vi "TCPIPmain.vi"(6 "data":T1(array[cluster]), 7 "config":T2, 8 "error in":errorcluster, 9 "data in":string, 10 "targer":enum16{"主舱外回路", "主舱内回路", "实验舱外回路", "实验舱内回路"}(ring), 11 "Enum":T3) -> (0 "error out":errorcluster, 1 "LED":bool[](array[boolean]), 2 "data out":T1(array[cluster]), 3 "Data?":bool[](array[boolean]))   [LabVIEW 2011]
uses:
  TCPIP_enum.ctl
  TCPIPconfig.ctl
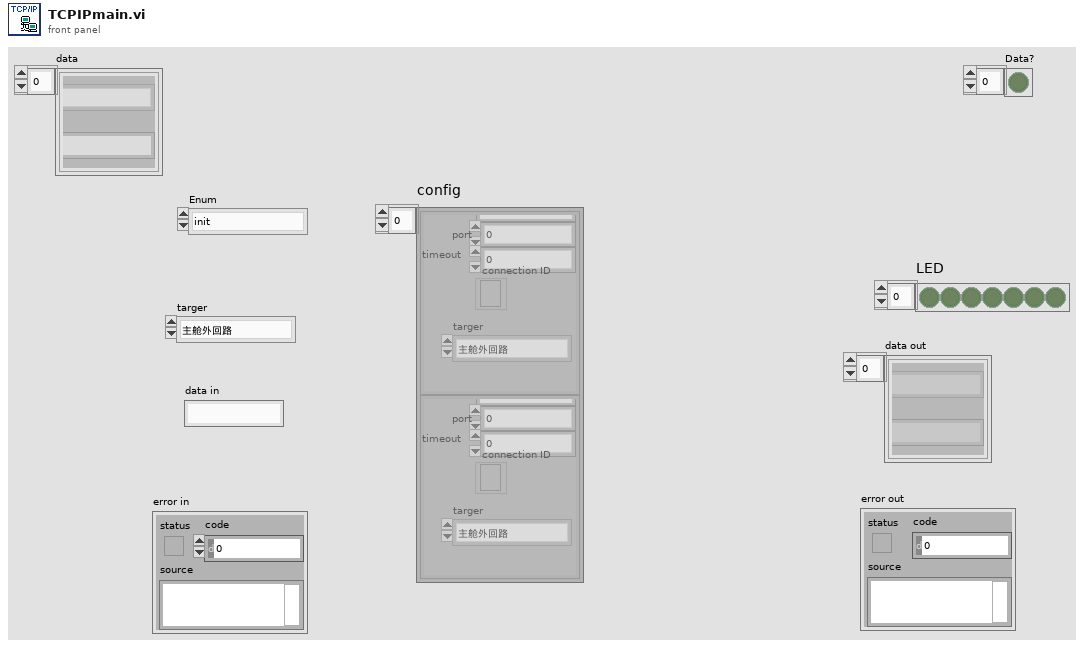
[diagram p1: front panel]
types:
  T1 = cluster{"targer":enum16{"主舱外回路", "主舱内回路", "实验舱外回路", "实验舱内回路"}, "data":string}[]
  T2 = typedef "TCPIPconfig.ctl" = cluster{"add":string, "port":u32, "timeout":u16, "connection ID":refnum<k5>, "targer":enum16{"主舱外回路", "主舱内回路", "实验舱外回路", "实验舱内回路"}}[]
  T3 = typedef "TCPIP_enum.ctl" = enum16{"init", "connect", "command", "write", "read", "close", "null"}
  T4 = cluster{"targer":enum16{"主舱外回路", "主舱内回路", "实验舱外回路", "实验舱内回路"}, "data":string}
  T5 = cluster{"add":string, "port":u32, "timeout":u16, "connection ID":refnum<k5>, "targer":enum16{"主舱外回路", "主舱内回路", "实验舱外回路", "实验舱内回路"}}
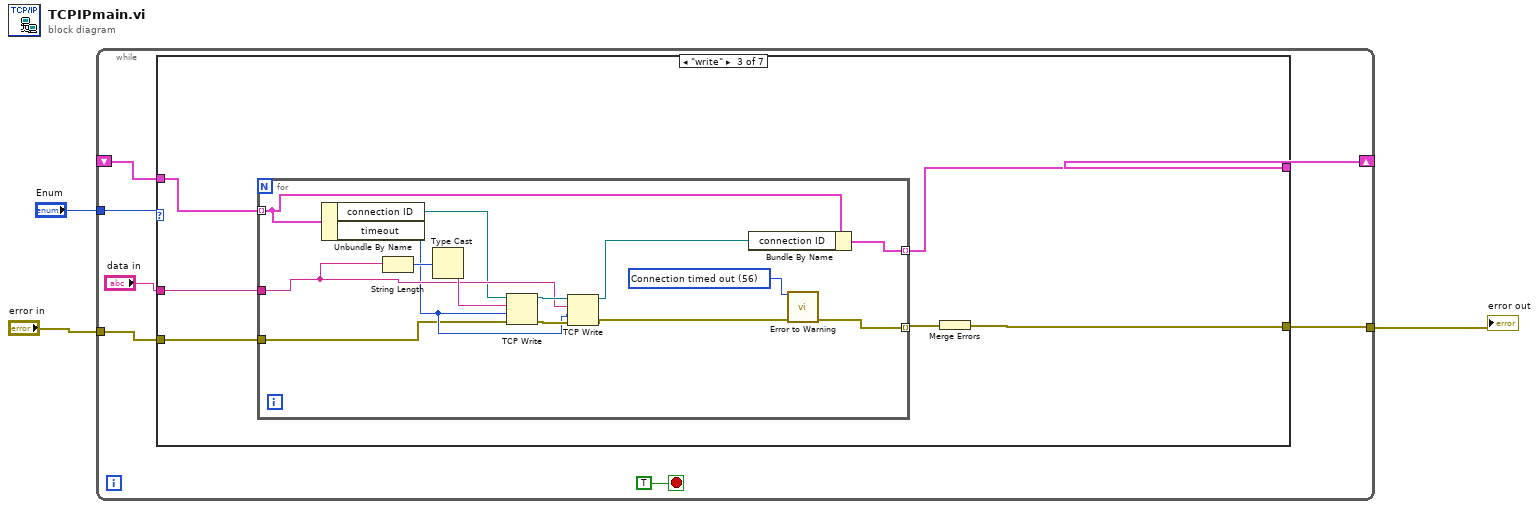
[diagram p0: block diagram]
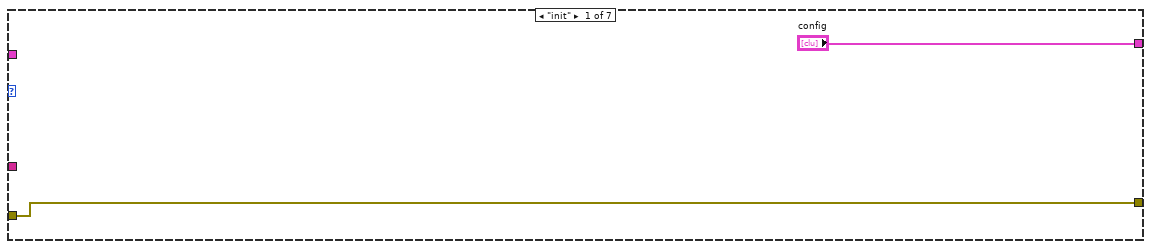
[diagram p2: hidden frame]
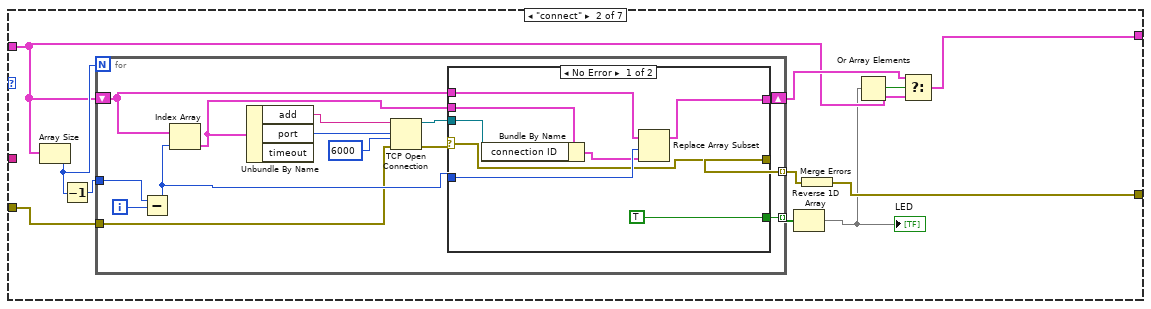
[diagram p3: hidden frame]
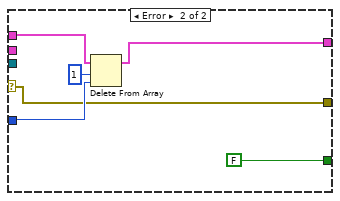
[diagram p4: hidden frame]
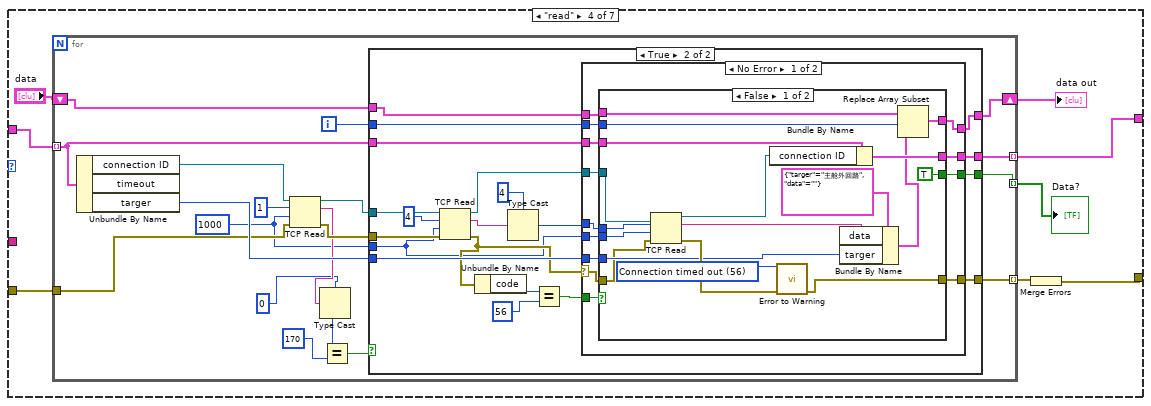
[diagram p5: hidden frame]
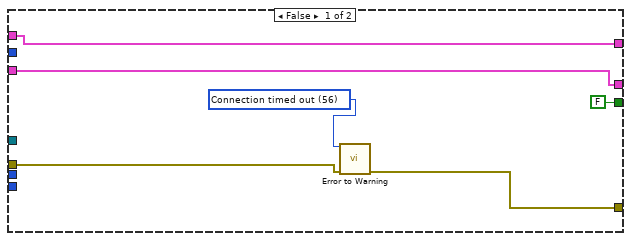
[diagram p6: hidden frame]
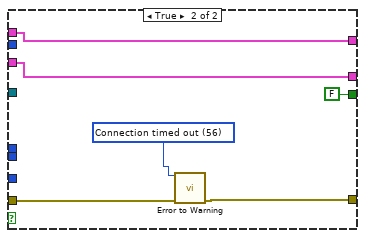
[diagram p7: hidden frame]
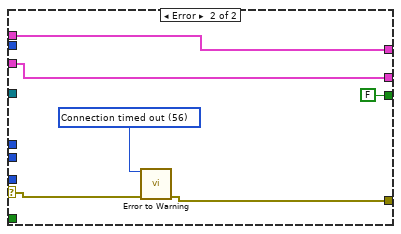
[diagram p8: hidden frame]
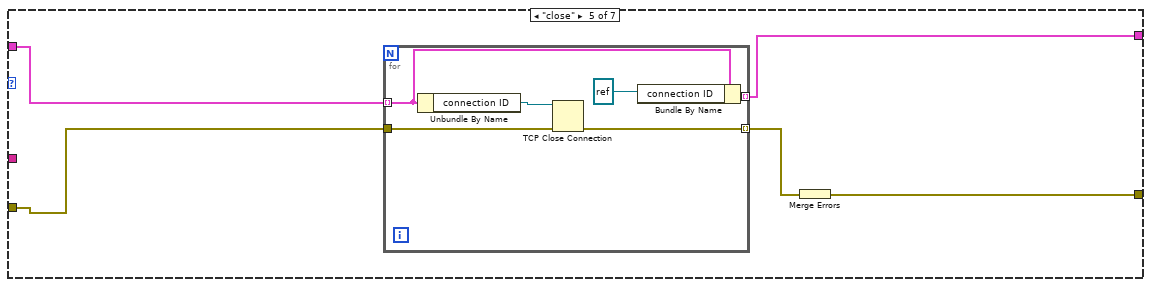
[diagram p9: hidden frame]
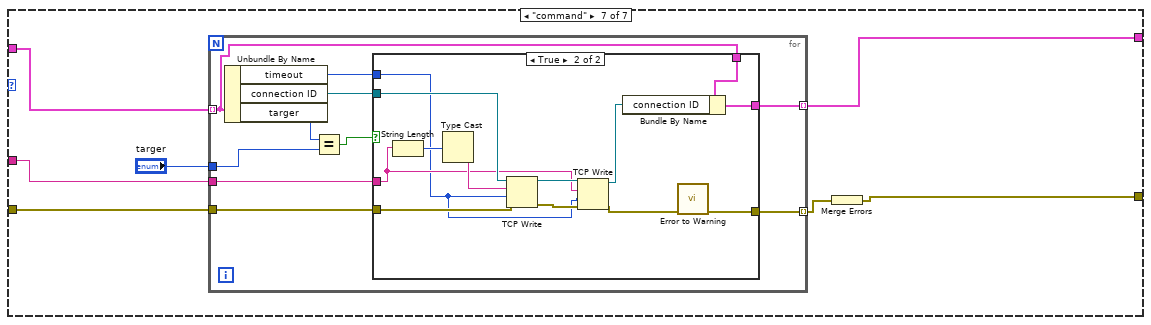
[diagram p11: hidden frame]
diagram:
  n1 = while {
    shift-right: [w8] -> _
    shift-left: _ -> [w7]
    tunnel: [w6] -> w2
    tunnel: "error in" -> [w5]
    tunnel: "Enum" -> [w9]
    stop <- TRUE stop-if-true
    n2 = case shown="\"write\"" w9 {
      tunnel: ["config" w14 w56 w78 w168 w180 w183] -> w8
      tunnel: w7 -> [_ w15 w57 w79 w172 w180 w187]
      tunnel: [w11 w20 w54 w76 w169 w179 w182] -> w6
      tunnel: w5 -> [w11 w22 w53 w75 w171 w179 w185]
      tunnel: "data in" -> [_ _ w52 _ _ _ w184]
      frame "init" {
      }
      frame "connect" {
        n3 = Array Size(array=w15) -> (size(s)=w19:i32)
        n4 = Decrement(x=w19) -> (x-1=w23:i32)
        n5 = for {
          N: w19 -> [_]
          shift-right: [w29] -> w16
          shift-left: w15 -> [w33]
          tunnel: w23 -> [w31]
          tunnel: w22 -> [w28]
          tunnel: [w27] -> w21 mode=indexing
          tunnel: [w26] -> w18 mode=indexing
          i -> [w32]
          n6 = Subtract(x=w31, y=w32) -> (x-y=w30:i32)
          n7 = Index Array(array=w33, index=w30) -> (element=w34:T5)
          n8 = Unbundle By Name(w34) -> ("add"=w37:string, "port"=w25:u32)  [unwired: 1 out]
          n9 = TCP Open Connection(address=w37, remote port or service name=w25, timeout ms (60000)=6000, error in (no error)=w28) -> (connection ID=w36:refnum<k5>, error out=w35:errorcluster)  [unwired: 1 in]
          n10 = case shown="No Error" w35 {
            selector: w35 -> [w39 w47]
            tunnel: w36 -> [w45 _]
            tunnel: w34 -> [w44 _]
            tunnel: w33 -> [w43 w51]
            tunnel: w30 -> [w42 w49]
            tunnel: [w40 w48] -> w29
            tunnel: [w39 w47] -> w27
            tunnel: [TRUE FALSE] -> w26
            frame No Error {
              n11 = Bundle By Name(cluster=w44, "connection ID"=w45) -> (w41:T5)
              n12 = Replace Array Subset "Replace Array Subset"(array=w43, new element=w41, index=w42) -> (w40:T2)
            }
            frame Error {
              n13 = Delete From Array(array=w51, length=1, index=w49) -> (array with subset deleted=w48:T2)  [unwired: 1 out]
            }
          }
        }
        n14 = Reverse 1D Array(array=w18) -> (reversed array=w13:bool[])
        "LED" <- w13
        n15 = Merge Errors(w21) -> (w20:errorcluster)
        n16 = Or Array Elements(Boolean array=w13) -> (logical OR=w17:bool)
        n17 = Select(t=w16, s=w17, f=w15) -> (s? t:f=w14:T2)
      }
      frame "write" {
        n18 = for {
          tunnel: w57 -> [w63] mode=indexing
          tunnel: w52 -> [w66]
          tunnel: [w61] -> w56 mode=indexing
          tunnel: [w60] -> w55 mode=indexing
          tunnel: w53 -> [w59]
          w58 = 56 items=["No Error", "Argument Error", "Memory Full", "Out of Zone", "End of File", "File Already Open", "Generic File IO Error", "File Not Found", "File Permission Error", "Disk Full", "Duplicate Path", "Too Many Files Open", "Not Enabled", "Resource File Not Found", "Cannot Add Resource", "Resource Not Found", "Image Not Found", "Image Memory Error", "Pen Does Not Exist", "Config Bad Type", "Config Token Not Found", "Config Parse Error", "Config Memory Error", "Bad External Code Format", "Bad External Code Offset", "External Code Not Present", "Null Window", "Destroy Window Mixup", "Null Menu", "Print Aborted", "Bad Print Record", "Print Driver Error", "Windows Error During Print", "Memory Error During Print", "Print Dialog Error", "Generic Print Error", "Invalid Device Refnum", "Device Not Found", "Device Parameter Error", "Device Unit Error", "Can't Open Device", "Device Call Aborted", "Generic Error", "Cancelled By User", "Object ID Too Low", "Object ID Too High", "Object Not In Heap", "Unknown Heap", "Bad DefProc ID", "DefProc Not In Table", "Message Out Of Range", "Null Method", "Unknown Message", "Manager Call Not Supported", "Bad address", "Connection In progress", "Connection timed out", "Connection is already in progress", "Network attribute not supported", "Network error", "Address in use", "System out of memory", "Connection aborted", "Connection refused", "Connection is not connected", "Connection is already connected", "Connection closed", "Initialize error (interapplication manager)", "Bad occurrence", "Wait on unbound occurrence handler", "Occurrence queue overflow", "Bad path", "Semaphore not signaled", "Unrecognized type (interapplication manager)"] ("1st Error to Convert")
          n19 = Unbundle By Name(w63) -> ("connection ID"=w65:refnum<k5>, "timeout"=w64:u16)
          n20 = String Length(string=w66) -> (length=w71:i32)
          n21 = Type Cast(x=w71) -> (*(type *) &x=w68:string)  [unwired: 1 out]
          n22 = TCP Write(connection ID=w65, data in=w68, error in (no error)=w59, 9:w64) -> (connection ID out=w70:refnum<k5>, error out=w69:errorcluster)  [unwired: 1 out]
          n23 = TCP Write(connection ID=w70, data in=w66, error in (no error)=w69, 9:w64) -> (connection ID out=w62:refnum<k5>, error out=w67:errorcluster)  [unwired: 1 out]
          n24 = Bundle By Name(cluster=w63, "connection ID"=w62) -> (w61:T5)
          n25 = call <vilib>:"Error to Warning.vi"("1st Error to Convert"=w58, "error in"=w67) -> ("warning out"=w60:errorcluster)  [unwired: 4 in, 9 out]
        }
        n26 = Merge Errors(w55) -> (w54:errorcluster)
      }
      frame "read" {
        n27 = for {
          tunnel: w79 -> [w98] mode=indexing
          tunnel: [w97] -> w78 mode=indexing
          tunnel: [w96] -> w77 mode=indexing
          tunnel: w75 -> [w94]
          shift-right: [w83] -> w73
          shift-left: "data" -> [w84]
          tunnel: [w81] -> w72 mode=indexing
          i -> [w82]
          w80 = 1000 ("timeout ms (25000)")
          n28 = Unbundle By Name(w98) -> ("connection ID"=w93:refnum<k5>, "targer"=w95:enum16{"主舱外回路", "主舱内回路", "实验舱外回路", "实验舱内回路"})  [unwired: 1 out]
          n29 = TCP Read(connection ID=w93, bytes to read=1, error in (no error)=w94, 9:w80) -> (connection ID out=w90:refnum<k5>, data out=w89:string, error out=w91:errorcluster)  [unwired: 1 out]
          n30 = Type Cast(type=u8 0, x=w89) -> (*(type *) &x=w87:u8)
          n31 = Equal?(x=w87, y=u8 170) -> (x = y?=w85:bool)
          n32 = case shown="True" w85 {
            tunnel: w90 -> [_ w120]
            tunnel: w98 -> [w104 w119]
            tunnel: [w104 w118] -> w97
            tunnel: [w100 w117] -> w96
            tunnel: w91 -> [w101 w116]
            tunnel: w95 -> [_ w115]
            tunnel: w80 -> [_ w109]
            tunnel: w84 -> [w103 w108]
            tunnel: [w103 w107] -> w83
            tunnel: w82 -> [_ w106]
            tunnel: [FALSE w105] -> w81
            frame False {
              w99 = 56 items=["No Error", "Argument Error", "Memory Full", "Out of Zone", "End of File", "File Already Open", "Generic File IO Error", "File Not Found", "File Permission Error", "Disk Full", "Duplicate Path", "Too Many Files Open", "Not Enabled", "Resource File Not Found", "Cannot Add Resource", "Resource Not Found", "Image Not Found", "Image Memory Error", "Pen Does Not Exist", "Config Bad Type", "Config Token Not Found", "Config Parse Error", "Config Memory Error", "Bad External Code Format", "Bad External Code Offset", "External Code Not Present", "Null Window", "Destroy Window Mixup", "Null Menu", "Print Aborted", "Bad Print Record", "Print Driver Error", "Windows Error During Print", "Memory Error During Print", "Print Dialog Error", "Generic Print Error", "Invalid Device Refnum", "Device Not Found", "Device Parameter Error", "Device Unit Error", "Can't Open Device", "Device Call Aborted", "Generic Error", "Cancelled By User", "Object ID Too Low", "Object ID Too High", "Object Not In Heap", "Unknown Heap", "Bad DefProc ID", "DefProc Not In Table", "Message Out Of Range", "Null Method", "Unknown Message", "Manager Call Not Supported", "Bad address", "Connection In progress", "Connection timed out", "Connection is already in progress", "Network attribute not supported", "Network error", "Address in use", "System out of memory", "Connection aborted", "Connection refused", "Connection is not connected", "Connection is already connected", "Connection closed", "Initialize error (interapplication manager)", "Bad occurrence", "Wait on unbound occurrence handler", "Occurrence queue overflow", "Bad path", "Semaphore not signaled", "Unrecognized type (interapplication manager)"] ("1st Error to Convert")
              n33 = call <vilib>:"Error to Warning.vi"("1st Error to Convert"=w99, "error in"=w101) -> ("warning out"=w100:errorcluster)  [unwired: 4 in, 9 out]
            }
            frame True {
              n34 = TCP Read(connection ID=w120, bytes to read=4, error in (no error)=w116, 9:w109) -> (connection ID out=w123:refnum<k5>, data out=w124:string, error out=w110:errorcluster)  [unwired: 1 out]
              n35 = Unbundle By Name(w110) -> ("code"=w113:i32)
              n36 = Type Cast(type=4, x=w124) -> (*(type *) &x=w122:i32)
              n37 = Equal?(x=w113, y=56) -> (x = y?=w111:bool)
              n38 = case shown="No Error" w110 {
                selector: w110 -> [w125 w164]
                tunnel: w123 -> [w137 _]
                tunnel: w122 -> [w136 _]
                tunnel: w119 -> [w135 w167]
                tunnel: [w134 w167] -> w118
                tunnel: [w133 w163] -> w117
                tunnel: w115 -> [w132 _]
                tunnel: w111 -> [w131 _]
                tunnel: w109 -> [w130 _]
                tunnel: w108 -> [w129 w166]
                tunnel: [w128 w166] -> w107
                tunnel: w106 -> [w127 _]
                tunnel: [w126 FALSE] -> w105
                frame No Error {
                  n39 = case shown="False" w131 {
                    tunnel: w137 -> [w155 _]
                    tunnel: w136 -> [w154 _]
                    tunnel: w130 -> [w151 _]
                    tunnel: w135 -> [w150 w161]
                    tunnel: [w149 w161] -> w134
                    tunnel: [w147 w158] -> w133
                    tunnel: w132 -> [w144 _]
                    tunnel: w129 -> [w143 w160]
                    tunnel: [w142 w160] -> w128
                    tunnel: w127 -> [w140 _]
                    tunnel: [TRUE FALSE] -> w126
                    tunnel: w125 -> [w138 w156]
                    frame False {
                      w152 = 56 items=["No Error", "Argument Error", "Memory Full", "Out of Zone", "End of File", "File Already Open", "Generic File IO Error", "File Not Found", "File Permission Error", "Disk Full", "Duplicate Path", "Too Many Files Open", "Not Enabled", "Resource File Not Found", "Cannot Add Resource", "Resource Not Found", "Image Not Found", "Image Memory Error", "Pen Does Not Exist", "Config Bad Type", "Config Token Not Found", "Config Parse Error", "Config Memory Error", "Bad External Code Format", "Bad External Code Offset", "External Code Not Present", "Null Window", "Destroy Window Mixup", "Null Menu", "Print Aborted", "Bad Print Record", "Print Driver Error", "Windows Error During Print", "Memory Error During Print", "Print Dialog Error", "Generic Print Error", "Invalid Device Refnum", "Device Not Found", "Device Parameter Error", "Device Unit Error", "Can't Open Device", "Device Call Aborted", "Generic Error", "Cancelled By User", "Object ID Too Low", "Object ID Too High", "Object Not In Heap", "Unknown Heap", "Bad DefProc ID", "DefProc Not In Table", "Message Out Of Range", "Null Method", "Unknown Message", "Manager Call Not Supported", "Bad address", "Connection In progress", "Connection timed out", "Connection is already in progress", "Network attribute not supported", "Network error", "Address in use", "System out of memory", "Connection aborted", "Connection refused", "Connection is not connected", "Connection is already connected", "Connection closed", "Initialize error (interapplication manager)", "Bad occurrence", "Wait on unbound occurrence handler", "Occurrence queue overflow", "Bad path", "Semaphore not signaled", "Unrecognized type (interapplication manager)"] ("1st Error to Convert")
                      n40 = TCP Read(connection ID=w155, bytes to read=w154, error in (no error)=w138, 9:w151) -> (connection ID out=w148:refnum<k5>, data out=w145:string, error out=w153:errorcluster)  [unwired: 1 out]
                      n41 = Bundle By Name(cluster=w150, "connection ID"=w148) -> (w149:T5)
                      n42 = call <vilib>:"Error to Warning.vi"("1st Error to Convert"=w152, "error in"=w153) -> ("warning out"=w147:errorcluster)  [unwired: 4 in, 9 out]
                      n43 = Bundle By Name(cluster=T4 {"targer"=enum."主舱外回路", "data"=""} ("data out"), "data"=w145, "targer"=w144) -> (w141:T4)
                      n44 = Replace Array Subset(array=w143, new element=w141, index=w140) -> (w142:T1)
                    }
                    frame True {
                      w157 = 56 items=["No Error", "Argument Error", "Memory Full", "Out of Zone", "End of File", "File Already Open", "Generic File IO Error", "File Not Found", "File Permission Error", "Disk Full", "Duplicate Path", "Too Many Files Open", "Not Enabled", "Resource File Not Found", "Cannot Add Resource", "Resource Not Found", "Image Not Found", "Image Memory Error", "Pen Does Not Exist", "Config Bad Type", "Config Token Not Found", "Config Parse Error", "Config Memory Error", "Bad External Code Format", "Bad External Code Offset", "External Code Not Present", "Null Window", "Destroy Window Mixup", "Null Menu", "Print Aborted", "Bad Print Record", "Print Driver Error", "Windows Error During Print", "Memory Error During Print", "Print Dialog Error", "Generic Print Error", "Invalid Device Refnum", "Device Not Found", "Device Parameter Error", "Device Unit Error", "Can't Open Device", "Device Call Aborted", "Generic Error", "Cancelled By User", "Object ID Too Low", "Object ID Too High", "Object Not In Heap", "Unknown Heap", "Bad DefProc ID", "DefProc Not In Table", "Message Out Of Range", "Null Method", "Unknown Message", "Manager Call Not Supported", "Bad address", "Connection In progress", "Connection timed out", "Connection is already in progress", "Network attribute not supported", "Network error", "Address in use", "System out of memory", "Connection aborted", "Connection refused", "Connection is not connected", "Connection is already connected", "Connection closed", "Initialize error (interapplication manager)", "Bad occurrence", "Wait on unbound occurrence handler", "Occurrence queue overflow", "Bad path", "Semaphore not signaled", "Unrecognized type (interapplication manager)"] ("1st Error to Convert")
                      n45 = call <vilib>:"Error to Warning.vi"("1st Error to Convert"=w157, "error in"=w156) -> ("warning out"=w158:errorcluster)  [unwired: 4 in, 9 out]
                    }
                  }
                }
                frame Error {
                  w162 = 56 items=["No Error", "Argument Error", "Memory Full", "Out of Zone", "End of File", "File Already Open", "Generic File IO Error", "File Not Found", "File Permission Error", "Disk Full", "Duplicate Path", "Too Many Files Open", "Not Enabled", "Resource File Not Found", "Cannot Add Resource", "Resource Not Found", "Image Not Found", "Image Memory Error", "Pen Does Not Exist", "Config Bad Type", "Config Token Not Found", "Config Parse Error", "Config Memory Error", "Bad External Code Format", "Bad External Code Offset", "External Code Not Present", "Null Window", "Destroy Window Mixup", "Null Menu", "Print Aborted", "Bad Print Record", "Print Driver Error", "Windows Error During Print", "Memory Error During Print", "Print Dialog Error", "Generic Print Error", "Invalid Device Refnum", "Device Not Found", "Device Parameter Error", "Device Unit Error", "Can't Open Device", "Device Call Aborted", "Generic Error", "Cancelled By User", "Object ID Too Low", "Object ID Too High", "Object Not In Heap", "Unknown Heap", "Bad DefProc ID", "DefProc Not In Table", "Message Out Of Range", "Null Method", "Unknown Message", "Manager Call Not Supported", "Bad address", "Connection In progress", "Connection timed out", "Connection is already in progress", "Network attribute not supported", "Network error", "Address in use", "System out of memory", "Connection aborted", "Connection refused", "Connection is not connected", "Connection is already connected", "Connection closed", "Initialize error (interapplication manager)", "Bad occurrence", "Wait on unbound occurrence handler", "Occurrence queue overflow", "Bad path", "Semaphore not signaled", "Unrecognized type (interapplication manager)"] ("1st Error to Convert")
                  n46 = call <vilib>:"Error to Warning.vi"("1st Error to Convert"=w162, "error in"=w164) -> ("warning out"=w163:errorcluster)  [unwired: 4 in, 9 out]
                }
              }
            }
          }
        }
        "data out" <- w73
        "Data?" <- w72
        n47 = Merge Errors(w77) -> (w76:errorcluster)
      }
      frame "close" {
        n48 = for {
          tunnel: w172 -> [w175] mode=indexing
          tunnel: w171 -> [w177]
          tunnel: [w176] -> w170 mode=indexing
          tunnel: [w173] -> w168 mode=indexing
          n49 = Unbundle By Name(w175) -> ("connection ID"=w178:refnum<k5>)
          n50 = TCP Close Connection(connection ID=w178, error in (no error)=w177) -> (error out=w176:errorcluster)  [unwired: 2 out]
          n51 = Bundle By Name(cluster=w175, "connection ID"=refnum<k5> refnum) -> (w173:T5)
        }
        n52 = Merge Errors(w170) -> (w169:errorcluster)
      }
      frame "null", Default {
      }
      frame "command" {
        n53 = for {
          tunnel: w187 -> [w189] mode=indexing
          tunnel: "targer" -> [w196]
          tunnel: w185 -> [w193]
          tunnel: [w192] -> w181 mode=indexing
          tunnel: w184 -> [w191]
          tunnel: [w188] -> w183 mode=indexing
          n54 = Unbundle By Name(w189) -> ("timeout"=w190:u16, "connection ID"=w194:refnum<k5>, "targer"=w197:enum16{"主舱外回路", "主舱内回路", "实验舱外回路", "实验舱内回路"})
          n55 = Equal?(x=w197, y=w196) -> (x = y?=w195:bool)
          n56 = case shown="True" w195 {
            tunnel: w194 -> [_ w207]
            tunnel: w193 -> [w198 w206]
            tunnel: [w198 w205] -> w192
            tunnel: w191 -> [_ w204]
            tunnel: w190 -> [_ w203]
            tunnel: w189 -> [w199 w202]
            tunnel: [w199 w200] -> w188
            frame False {
            }
            frame True {
              n57 = String Length(string=w204) -> (length=w212:i32)
              n58 = Type Cast(x=w212) -> (*(type *) &x=w209:string)  [unwired: 1 out]
              n59 = TCP Write(connection ID=w207, data in=w209, error in (no error)=w206, 9:w203) -> (connection ID out=w211:refnum<k5>, error out=w210:errorcluster)  [unwired: 1 out]
              n60 = TCP Write(connection ID=w211, data in=w204, error in (no error)=w210, 9:w203) -> (connection ID out=w201:refnum<k5>, error out=w208:errorcluster)  [unwired: 1 out]
              n61 = Bundle By Name(cluster=w202, "connection ID"=w201) -> (w200:T5)
              n62 = call <vilib>:"Error to Warning.vi"("error in"=w208) -> ("warning out"=w205:errorcluster)  [unwired: 5 in, 9 out]
            }
          }
        }
        n63 = Merge Errors(w181) -> (w182:errorcluster)
      }
    }
  }
  "error out" <- w2
